vi "Kick Error Histogram.vi"(11 "IA state":T1={"our_robots"=[], "enemy_robots"=[], "balls"=[], "geometry"={"line_width"=0, "field_length"=0, "field_width"=0, "boundary_width"=0, "referee_width"=0, "goal_width"=0, "goal_depth"=0, "goal_wall_width"=0, "center_circle_radius"=0, "defense_radius"=0, "defense_stretch"=0, "free_kick_from_defense_dist"=0, "penalty_spot_from_field_line_dist"=0, "penalty_line_from_spot_dist"=0}, "IA Judge"={"stage"="", "command"="", "our_goalie_id"=0.0, "enemy_goalie_id"=0.0, "command enum"=enum."Halt", "Time"=enum."Azul"}, "Received Timestamp"=timestamp(0 s since 1904-01-01), "Events"={"Touch"=FALSE, "Ball out"=FALSE, "id touch"=0.0, "Ball out of \nVision"=FALSE, "Ball inside \nGoalie area"=FALSE, "Robot not responding"=FALSE, "Robots responding status"=[1.0, 1.0, 1.0, 1.0, 1.0, 1.0], "Enemy Ball \nPossession"=FALSE, "Pass State"=FALSE, "id end of pass"=0.0, "Kick"=FALSE, "Id ini Possession"=0.0, "Ball Possesion"=FALSE, "Id Possesion"=0.0}}) -> (3 "Kick Error Histogram":cluster{dbl[], dbl[]}(graph))   [LabVIEW 2017]
uses:
  Core/AI Input.ctl
  Core/AI Robot.ctl
  Intel/Functions Enum.ctl
  Intel/AttackerStates.ctl
  Core/AI Ball.ctl
  Core/Field Size.ctl
  Core/AI Judge.ctl
  Intel/Command Enum.ctl
  Util/Events/Events.ctl
panel:
  out "Array":dbl[](array[numeric])
  in  "Divisões do gol":i32=14
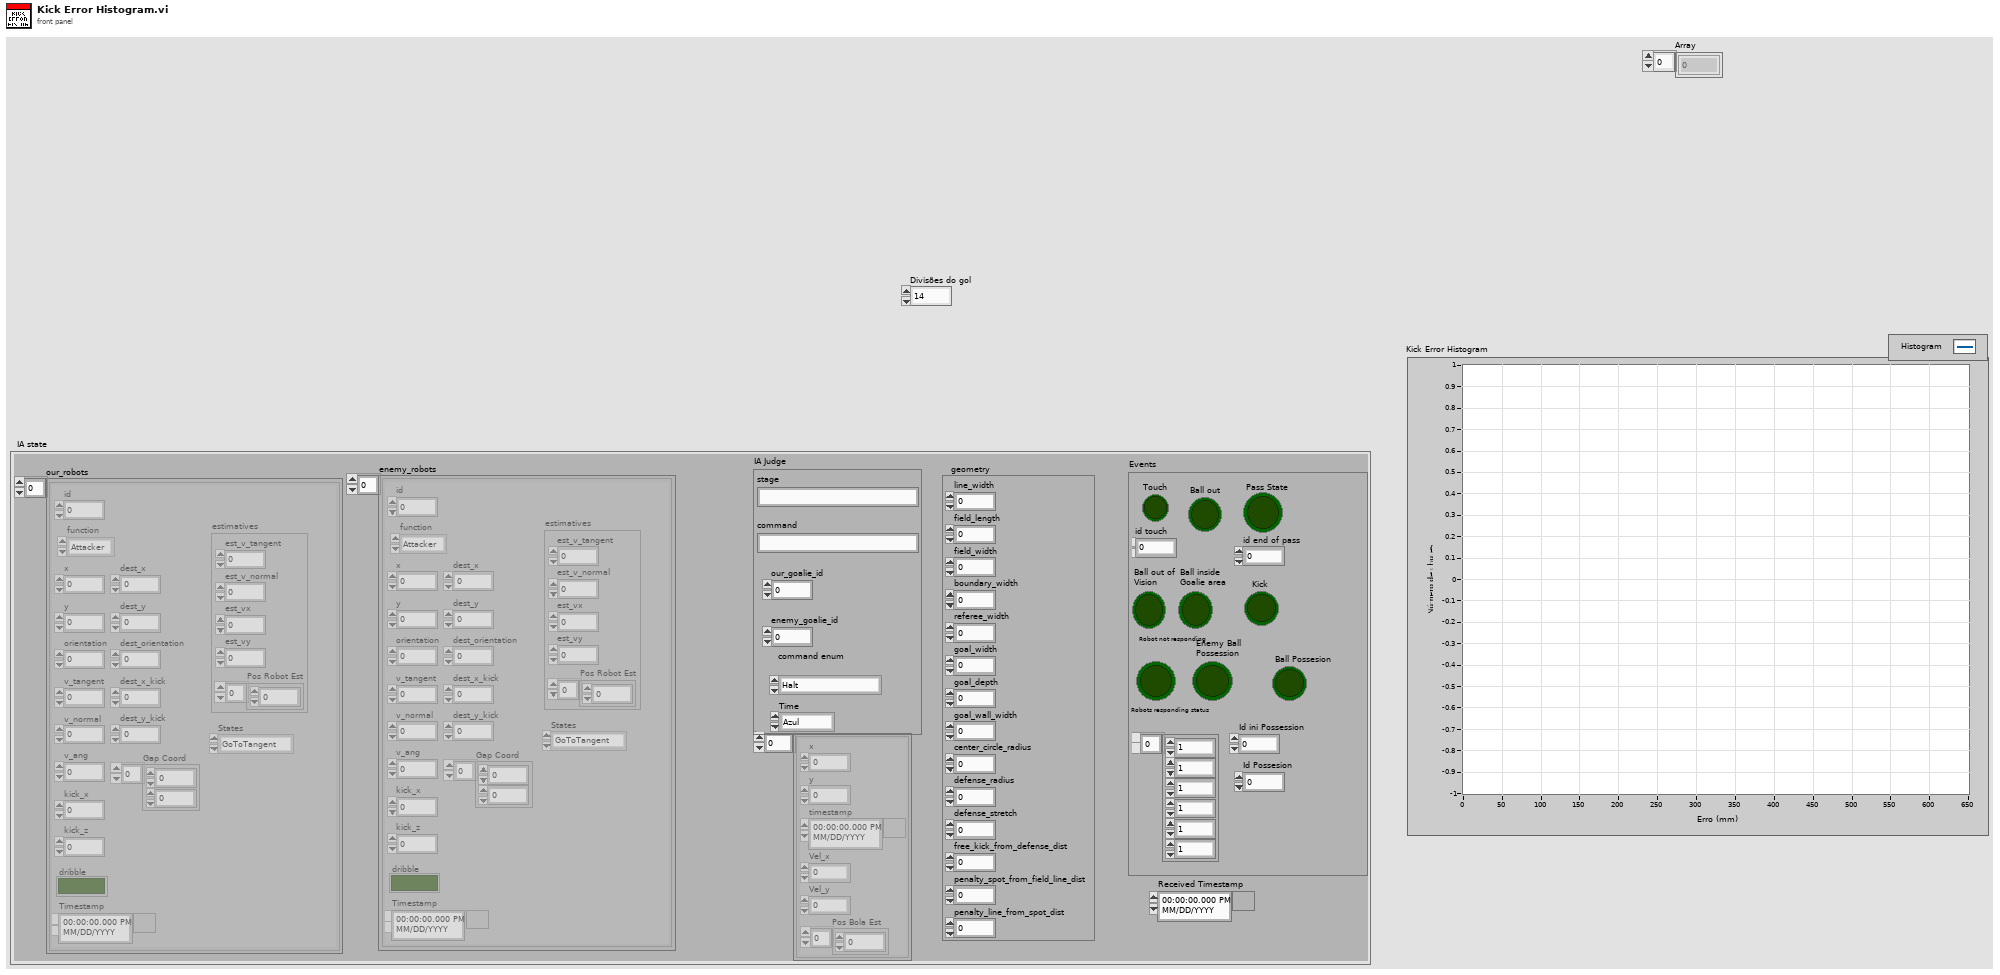
[diagram p1: front panel]
types:
  T1 = typedef "AI Input.ctl" = cluster{"our_robots":T2[], "enemy_robots":T2[], "balls":T5[], "geometry":T6, "IA Judge":T7, "Received Timestamp":timestamp, "Events":T9}
  T2 = typedef "AI Robot.ctl" = cluster{"id":u32, "function":T3, "x":dbl, "y":dbl, "orientation":dbl, "v_tangent":dbl, "v_normal":dbl, "v_ang":dbl, "kick_x":dbl, "kick_z":dbl, "dribble":bool, "Timestamp":timestamp, "dest_x":dbl, "dest_y":dbl, "dest_orientation":dbl, "estimatives":cluster{"est_v_tangent":dbl, "est_v_normal":dbl, "est_vx":dbl, "est_vy":dbl, "Pos Robot Est":dbl[]}, "dest_x_kick":dbl, "dest_y_kick":dbl, "Gap Coord":dbl[], "States":T4}
  T3 = typedef "Functions Enum.ctl" = enum16{"Attacker", "Goalie", "Defender", "Striker", "Goto 0", "Dummy", "Kicker", "ZigZag"}
  T4 = typedef "AttackerStates.ctl" = enum16{"Pass", "GoToTangent", "BallGetting", "GoToKick", ""}
  T5 = typedef "AI Ball.ctl" = cluster{"x":dbl, "y":dbl, "timestamp":timestamp, "Vel_x":dbl, "Vel_y":dbl, "Pos Bola Est":dbl[]}
  T6 = typedef "Field Size.ctl" = cluster{"line_width":u32, "field_length":u32, "field_width":u32, "boundary_width":u32, "referee_width":u32, "goal_width":u32, "goal_depth":u32, "goal_wall_width":u32, "center_circle_radius":u32, "defense_radius":u32, "defense_stretch":u32, "free_kick_from_defense_dist":u32, "penalty_spot_from_field_line_dist":u32, "penalty_line_from_spot_dist":u32}
  T7 = typedef "AI Judge.ctl" = cluster{"stage":string, "command":string, "our_goalie_id":dbl, "enemy_goalie_id":dbl, "command enum":T8, "Time":enum16{"Azul", "Amarelo"}}
  T8 = typedef "Command Enum.ctl" = enum16{"Halt", "Stop", "Force Start", "PKA Normal Start", "Prepare Kickoff Ally", "PKE Normal Start", "Prepare Kickoff Enemy", "Prepare Penalty Ally", "PPA Normal Start", "Prepare Penalty Enemy", "PPE Normal Start", "Direct Free Enemy", "Direct Free Ally", "Indirect Free Enemy", "Indirect Free Ally", "Timeout Enemy", "Timeout Ally", "Goal Enemy", "Goal Ally", "Ball Placement Enemy", "Ball Placement Ally", "Normal Half Time", "Extra Time Break", "Extra Half Time", "None", "Post Game"}
  T9 = typedef "Events.ctl" = cluster{"Touch":bool, "Ball out":bool, "id touch":dbl, "Ball out of \nVision":bool, "Ball inside \nGoalie area":bool, "Robot not responding":bool, "Robots responding status":dbl[], "Enemy Ball \nPossession":bool, "Pass State":bool, "id end of pass":dbl, "Kick":bool, "Id ini Possession":dbl, "Ball Possesion":bool, "Id Possesion":dbl}
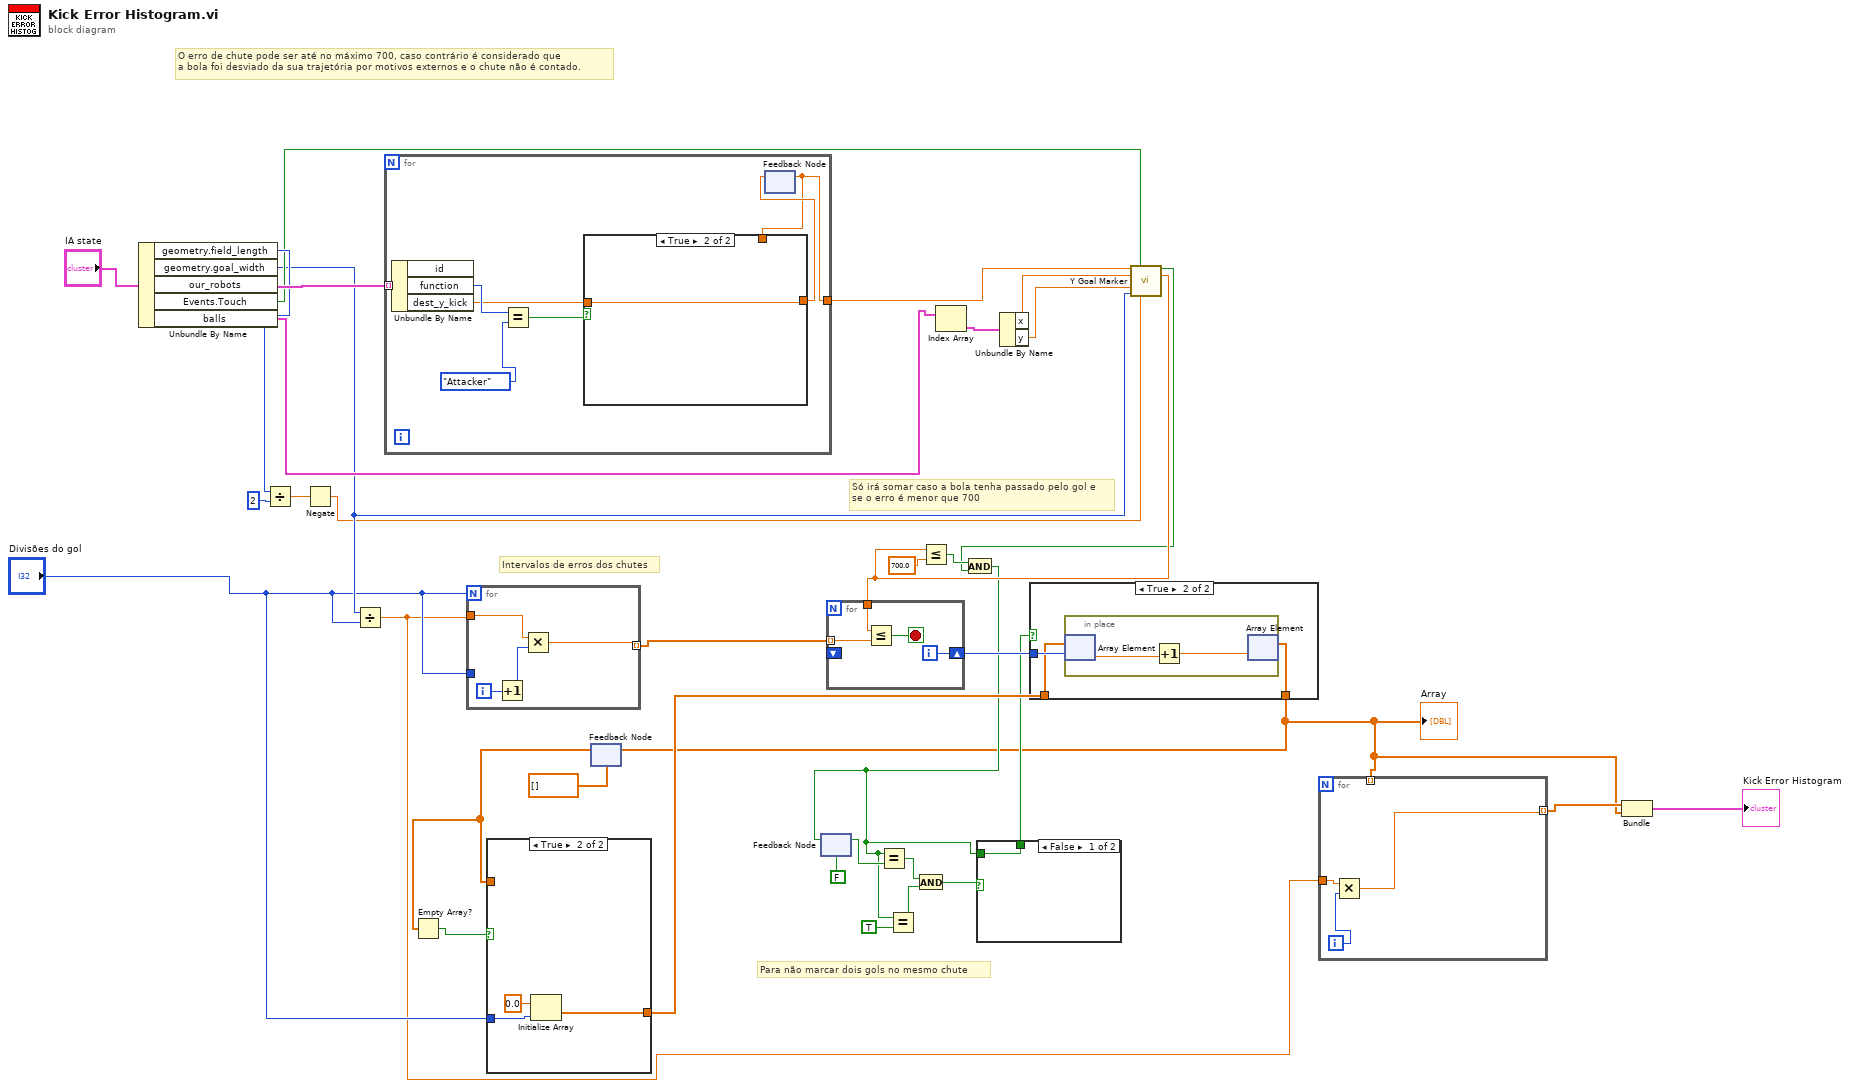
[diagram p0: block diagram]
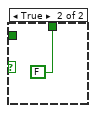
[diagram p2: hidden frame]
diagram:
  # "Para não marcar dois gols no mesmo chute"
  # "Só irá somar caso a bola tenha passado pelo gol e\nse o erro é menor que 700"
  # "Intervalos de erros dos chutes"
  # "O erro de chute pode ser até no máximo 700, caso contrário é considerado que\na bola foi desviado da sua trajetória por motivos externos e o chute não é contado."
  n1 = Unbundle By Name("IA state") -> ("geometry.field_length"=w34:u32, "geometry.goal_width"=w22:u32, "our_robots"=w35:T2[], "Events.Touch"=w24:bool, "balls"=w26:T5[])
  n2 = Divide(x=w34, y=u32 2) -> (x/y=w15:dbl)
  n3 = Negate(x=w15) -> (-x=w14:dbl)
  n4 = Divide(x=w22, y="Divisões do gol") -> (x/y=w1:dbl)
  n5 = for {
    tunnel: w35 -> [w43] mode=indexing
    tunnel: [w37] -> w23
    n6 = Unbundle By Name(w43) -> ("function"=w42:T3, "dest_y_kick"=w39:dbl)  [unwired: 1 out]
    n7 = Equal?(x=w42, y=Functions_Enum."Attacker" ("function")) -> (x = y?=w40:bool)
    n8 = feedback #1() -> (w37:dbl)  [unwired: 1 in]
    n9 = case shown="True" w40 {
      tunnel: [w44 w45] -> w38
      tunnel: w39 -> [_ w45]
      tunnel: w37 -> [w44 _]
      frame False {
      }
      frame True {
      }
    }
    n10 = feedback-in #1(w38) -> ()
  }
  n11 = for {
    N: "Divisões do gol" -> [_]
    tunnel: w1 -> [w49]
    tunnel: "Divisões do gol" -> [_]
    tunnel: [w48] -> w32 mode=indexing
    i -> [w47]
    n12 = Increment(x=w47) -> (x+1=w46:i32)
    n13 = Multiply(x=w49, y=w46) -> (x*y=w48:dbl)
  }
  n14 = feedback #2(dbl[] []) -> (w29:dbl[])
  n15 = Empty Array?(array=w29) -> (empty?=w28:bool)
  n16 = case shown="True" w28 {
    tunnel: w29 -> [w50 _]
    tunnel: [w50 w52] -> w27
    tunnel: "Divisões do gol" -> [_ w51]
    frame False {
    }
    frame True {
      n17 = Initialize Array(0.0 ("element"), w51) -> (w52:dbl[])
    }
  }
  n18 = feedback #3(FALSE) -> (w12:bool)
  n19 = Index Array(array=w26) -> (element=w25:T5)  [unwired: 1 in]
  n20 = Unbundle By Name(w25) -> ("x"=w20:dbl, "y"=w21:dbl)
  n21 = call "Y Goal Marker.vi"("dest_y_kick"=w23, "Touch"=w24, "ball x"=w20, "ball y"=w21, "goal width"=w22, "goal x"=w14) -> ("Goal or Not"=w16:bool, "kick error"=w19:dbl)  [unwired: 8 in]
  n22 = for {
    shift-right: [w56] -> w31
    shift-left: _ -> [_]
    tunnel: w32 -> [w55] mode=indexing
    tunnel: w19 -> [w54]
    i -> [w56]
    stop <- w57 stop-if-true
    n23 = Less Or Equal?(x=w54, y=w55) -> (x <= y?=w57:bool)
  }
  n24 = Less Or Equal?(x=w19, y=700.0) -> (x <= y?=w17:bool)
  n25 = And(x=w17, y=w16) -> (x .and. y?=w6:bool)
  n26 = feedback-in #3(w6) -> ()
  n27 = Equal?(x=w6, y=w12) -> (x = y?=w11:bool)
  n28 = Equal?(x=w6, y=TRUE) -> (x = y?=w9:bool)
  n29 = And(x=w11, y=w9) -> (x .and. y?=w8:bool)
  n30 = case shown="False" w8 {
    tunnel: [w58 FALSE] -> w7
    tunnel: w6 -> [w58 _]
    frame False {
    }
    frame True {
    }
  }
  n31 = case shown="True" w7 {
    tunnel: w31 -> [_ w63]
    tunnel: w27 -> [w60 w62]
    tunnel: [w60 w61] -> w4
    frame False {
    }
    frame True {
      n32 = in-place {
        n33 = in-place-array #4(w62, w63) -> (w65:dbl)
        n34 = Increment(x=w65) -> (x+1=w64:dbl)
        n35 = in-place-array #4(w64) -> (w61:dbl[])  [unwired: 1 out]
      }
    }
  }
  "Array" <- w4
  n36 = feedback-in #2(w4) -> ()
  n37 = for {
    tunnel: w4 -> [_] mode=indexing
    tunnel: [w67] -> w5 mode=indexing
    tunnel: w1 -> [w66]
    i -> [w68]
    n38 = Multiply(x=w66, y=w68) -> (x*y=w67:dbl)
  }
  n39 = Bundle(w5, w4) -> (→"Kick Error Histogram":cluster{dbl[], dbl[]})  [unwired: 1 in]
